vi "CamInit.vi"(8 "error in (no error)":errorcluster, 11 "Refnum in":T1) -> (0 "error out":errorcluster, 3 "Refnum out":T1)   [LabVIEW 2020]
uses:
  <vilib>/userDefined/High Color/IMAQdx.ctl
  <vilib>/vision/driver/NI_Vision_Acquisition_Software.lvlib
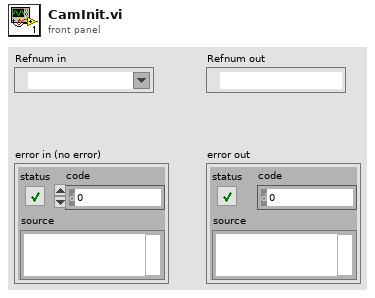
[diagram p1: front panel]
types:
  T1 = typedef "IMAQdx.ctl" = refnum<k21>
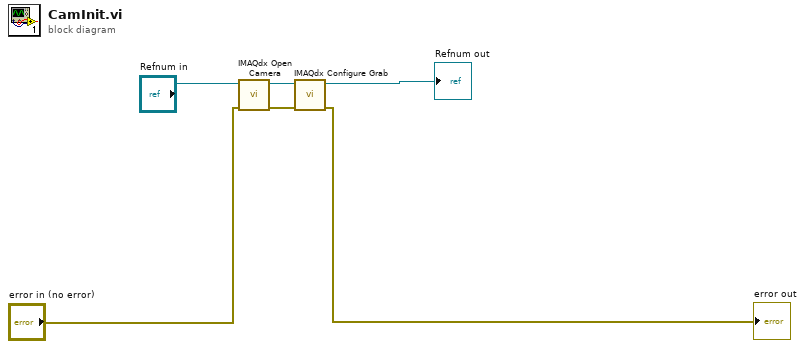
[diagram p0: block diagram]
diagram:
  n1 = call <vilib>:"IMAQdx Open Camera.vi"("error in"="error in (no error)", "Session In"="Refnum in") -> ("error out"=w2:errorcluster, "Session Out"=w1:T1)  [unwired: 8 in]
  n2 = call <vilib>:"IMAQdx Configure Grab.vi"("error in"=w2, "Session In"=w1) -> ("error out"=→"error out":errorcluster, "Session Out"=→"Refnum out":T1)  [unwired: 8 in]
